vi "ReadAllPositions.vi"(8 "error in (no error)":errorcluster, 11 "UI MotionStatus in":refnum<class "UI MotionStatus.lvclass">) -> (0 "error out":errorcluster, 1 "Positions, mm":sgl[](array[numeric]), 3 "UI MotionStatus out":refnum<class "UI MotionStatus.lvclass">)   [LabVIEW 2018, in "UI MotionStatus.lvclass"]
uses:
  UI MotionStatus.lvclass
  UI MotionStatus.lvclass/UI MotionStatus.ctl
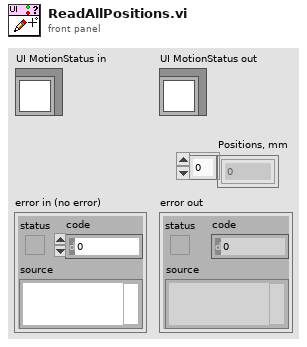
[diagram p1: front panel]
types:
  T1 = typedef "PositonIndicatorsCtrlRefs.ctl" = cluster{"BS1":refnum<vi>, "BS2":refnum<vi>, "BS3":refnum<vi>, "BS4":refnum<vi>, "RT3":refnum<vi>, "RT2":refnum<vi>, "RT1":refnum<vi>}
  T2 = typedef "MotionStatusLEDCtrlRefs.ctl" = cluster{"BS1":refnum<vi>, "BS2":refnum<vi>, "BS3":refnum<vi>, "BS4":refnum<vi>, "RT1":refnum<vi>, "RT2":refnum<vi>, "RT3":refnum<vi>}
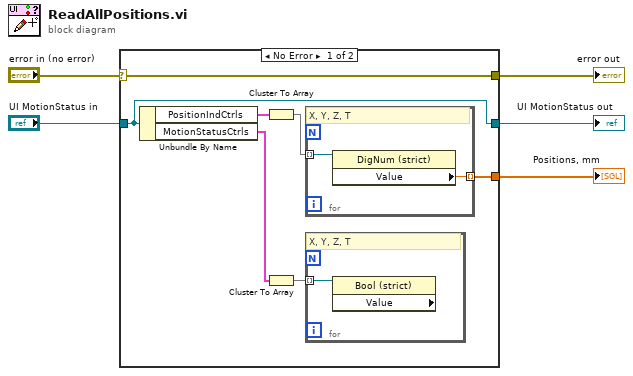
[diagram p0: block diagram]
diagram:
  n1 = case shown="No Error" "error in (no error)" {
    selector: "error in (no error)" -> [w12 w17]
    tunnel: [w12 w17] -> w4
    tunnel: [w10 w16] -> w2
    tunnel: "UI MotionStatus in" -> [w10 w16]
    tunnel: [w11 _] -> w1
    frame No Error {
      n2 = Unbundle By Name(w10) -> ("PositionIndCtrls"=w9:T1, "MotionStatusCtrls"=w7:T2)
      n3 = Cluster To Array(cluster=w9) -> (array=w8:refnum<vi>[])
      n4 = Cluster To Array(cluster=w7) -> (array=w6:refnum<vi>[])
      n5 = for {
        tunnel: [w14] -> w11 mode=indexing
        tunnel: w8 -> [w15] mode=indexing
        # "X, Y, Z, T"
        n6 = property class="DigNum (strict)"(reference=w15) -> ("Value"=w14:sgl)  [unwired: 1 in, 2 out]
      }
      n7 = for {
        tunnel: w6 -> [w13] mode=indexing
        # "X, Y, Z, T"
        n8 = property class="Bool (strict)" props=["Value"](reference=w13) -> ()  [unwired: 1 in, 3 out]
      }
    }
    frame Error {
    }
  }
  "error out" <- w4
  "UI MotionStatus out" <- w2
  "Positions, mm" <- w1
